vi "CTR_DataControlArrayConfigs.vi"(8 "error in":errorcluster, 11 "StreamCluster":T1={"DAQ_Configs"=[], "CTR_Config"={"CTR refDes"="", "CTR IP Addr"="", "Restart"=FALSE}, "Network_Configs"={"Buffer"=1, "ManagmentRate_Hz"=1000, "StreamRate_Hz"=10, "ConnectionHysterisis"=0, "LoggingRate_Hz"=10}, "ConfigXML_Checksum"=""}) -> (0 "error out":errorcluster={"status"=TRUE, "code"=0, "source"=""}, 3 "StreamCluster":T1)   [LabVIEW 2024]
uses:
  Control/CTR_ChannelList.ctl
  OneDrive - Embry-Riddle Aeronautical University/Admin/Facilities/TC3/TC3 DAC/Code/RTC_PXIe-Code v1_9_0 CODE/QMH-Architecture/support/Control/streamIO_states.ctl
  Control/CTR_StreamCluster_TypeDef.ctl
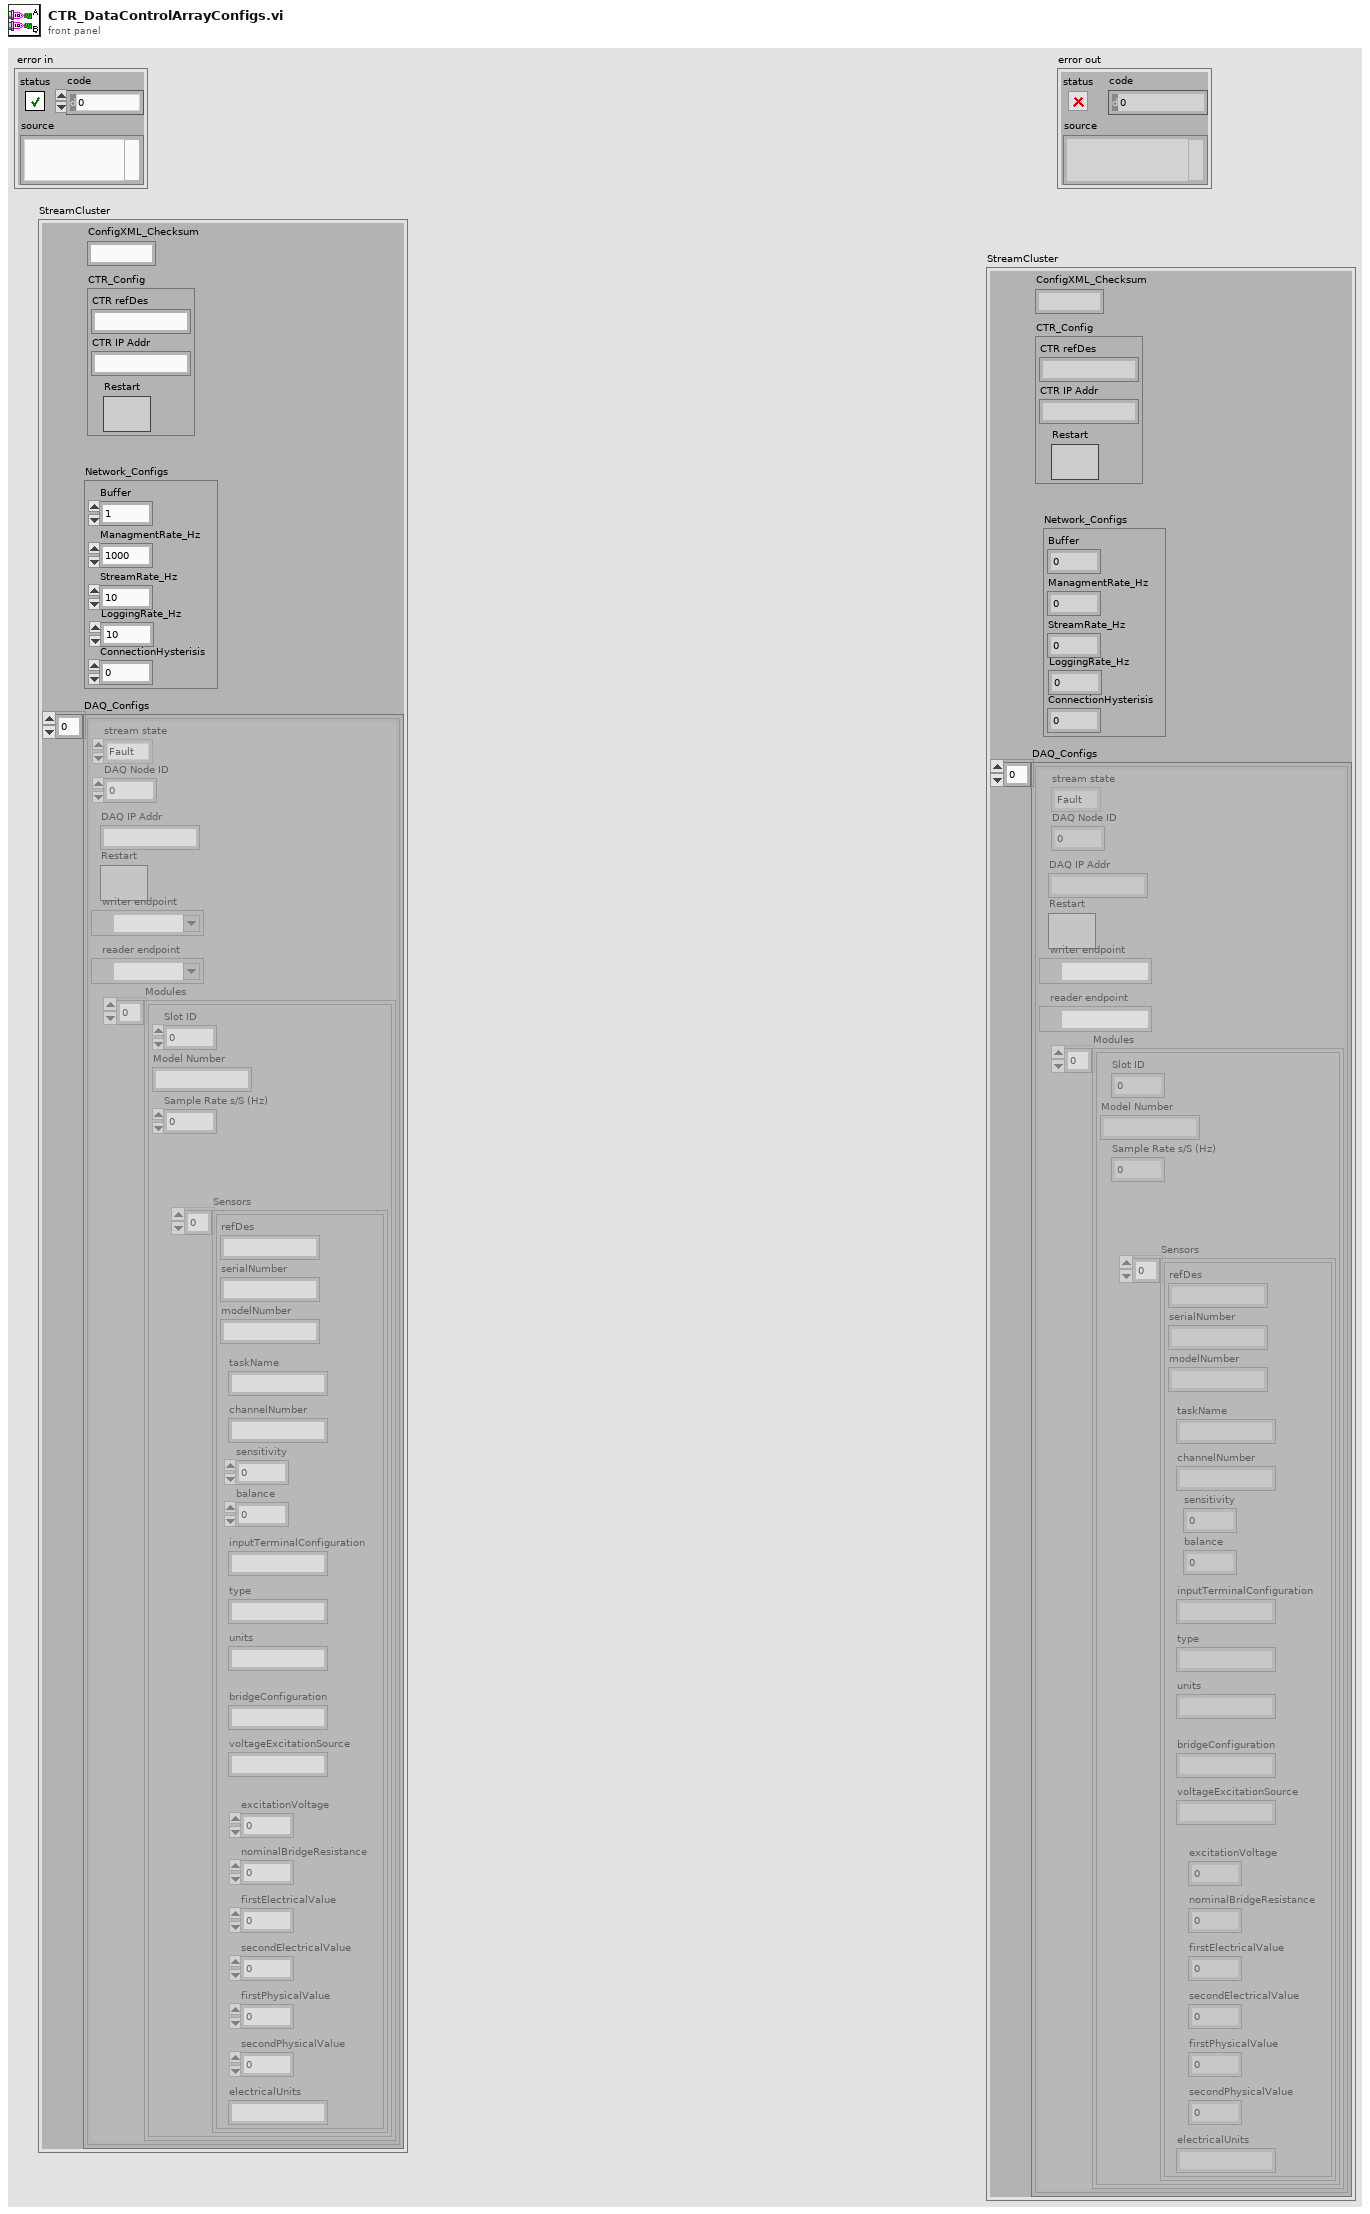
[diagram p1: front panel]
types:
  T1 = typedef "CTR_StreamCluster_TypeDef.ctl" = cluster{"DAQ_Configs":cluster{"stream state":T2, "DAQ Node ID":i32, "Modules":cluster{"Slot ID":i32, "Model Number":string, "Sample Rate s/S (Hz)":dbl, "Sensors":cluster{"refDes":string, "serialNumber":string, "modelNumber":string, "units":string, "balance":dbl, "sensitivity":dbl, "type":string, "inputTerminalConfiguration":string, "channelNumber":string, "taskName":string, "bridgeConfiguration":string, "excitationVoltage":dbl, "voltageExcitationSource":string, "nominalBridgeResistance":dbl, "firstElectricalValue":dbl, "secondElectricalValue":dbl, "firstPhysicalValue":dbl, "secondPhysicalValue":dbl, "electricalUnits":string}[]}[], "DAQ IP Addr":string, "Restart":bool, "writer endpoint":refnum<k21>, "reader endpoint":refnum<k21>}[], "CTR_Config":cluster{"CTR refDes":string, "CTR IP Addr":string, "Restart":bool}, "Network_Configs":cluster{"Buffer":i32, "ManagmentRate_Hz":i32, "StreamRate_Hz":i32, "ConnectionHysterisis":i32, "LoggingRate_Hz":i32}, "ConfigXML_Checksum":string}
  T2 = typedef "streamIO_states.ctl" = enum16{"Fault", "Initialize", "Stream", "Close"}
  T3 = typedef "CTR_ChannelList.ctl" = cluster{"CTR-refDes":string, "CTR-refDes-restart":string, "DAQs":cluster{"Channels":cluster{"refDes-sensor_parent":string, "refDes":string}[], "refDes-restart":string, "refDes-fault":string, "refDes-state":string, "refDes":string}[]}
  T4 = cluster{"stream state":T2, "DAQ Node ID":i32, "Modules":cluster{"Slot ID":i32, "Model Number":string, "Sample Rate s/S (Hz)":dbl, "Sensors":cluster{"refDes":string, "serialNumber":string, "modelNumber":string, "units":string, "balance":dbl, "sensitivity":dbl, "type":string, "inputTerminalConfiguration":string, "channelNumber":string, "taskName":string, "bridgeConfiguration":string, "excitationVoltage":dbl, "voltageExcitationSource":string, "nominalBridgeResistance":dbl, "firstElectricalValue":dbl, "secondElectricalValue":dbl, "firstPhysicalValue":dbl, "secondPhysicalValue":dbl, "electricalUnits":string}[]}[], "DAQ IP Addr":string, "Restart":bool, "writer endpoint":refnum<k21>, "reader endpoint":refnum<k21>}[]
  T5 = cluster{"Channels":cluster{"refDes-sensor_parent":string, "refDes":string}[], "refDes-restart":string, "refDes-fault":string, "refDes-state":string, "refDes":string}[]
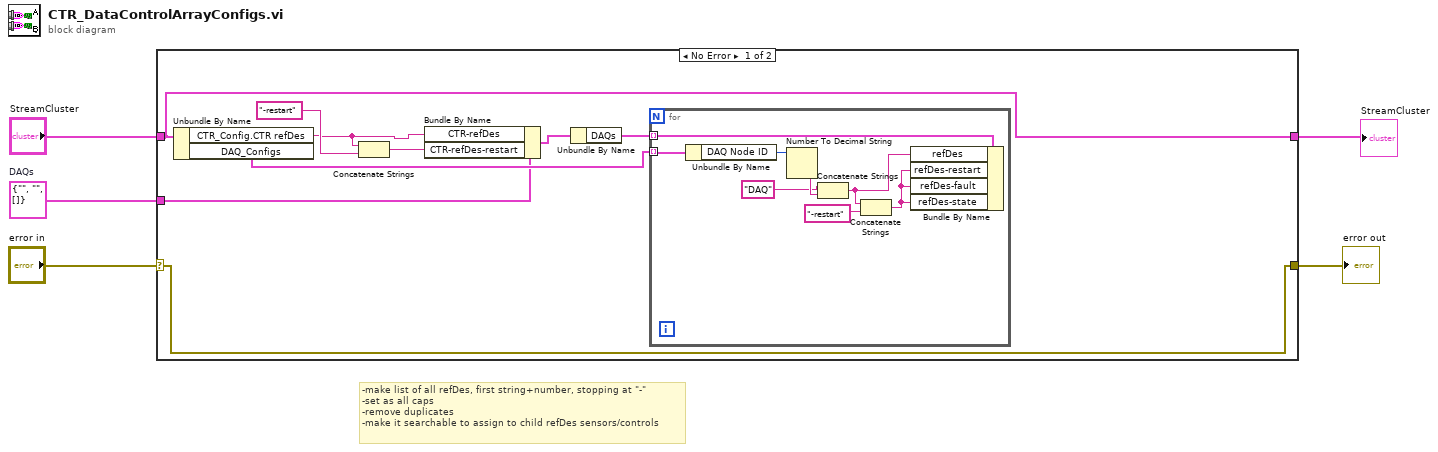
[diagram p0: block diagram]
diagram:
  w3 = T3 {"CTR-refDes"="", "CTR-refDes-restart"="", "DAQs"=[]}  # DAQs
  # "-make list of all refDes, first string+number, stopping at \"-\"\n-set as all caps\n-remove duplicates\n-make it searchable to assign to child refDes sensors/controls"
  n1 = case shown="No Error" "error in" {
    selector: "error in" -> [w7 w23]
    tunnel: [w7 w23] -> w4
    tunnel: [w6 w24] -> w1
    tunnel: "StreamCluster" -> [w6 w24]
    tunnel: w3 -> [w12 _]
    frame No Error {
      n2 = Unbundle By Name(w6) -> ("CTR_Config.CTR refDes"=w11:string, "DAQ_Configs"=w13:T4)
      n3 = Concatenate Strings(w11, "-restart" ("string")) -> (w10:string)
      n4 = Bundle By Name(cluster=w12, "CTR-refDes"=w11, "CTR-refDes-restart"=w10) -> (w9:T3)
      n5 = Unbundle By Name(w9) -> ("DAQs"=w8:T5)
      n6 = for {
        tunnel: w13 -> [w22] mode=indexing
        tunnel: w8 -> [w21] mode=indexing
        n7 = Unbundle By Name(w22) -> ("DAQ Node ID"=w20:i32)
        n8 = Number To Decimal String(number=w20) -> (decimal integer string=w19:string)  [unwired: 1 in]
        n9 = Concatenate Strings("DAQ" ("string"), w19) -> (w17:string)
        n10 = Concatenate Strings(w17, "-restart") -> (w15:string)
        n11 = Bundle By Name(cluster=w21, "refDes"=w17, "refDes-restart"=w15, "refDes-fault"=w15, "refDes-state"=w15) -> ()  [unwired: 1 out]
      }
    }
    frame Error {
    }
  }
  "error out" <- w4
  "StreamCluster" <- w1
